vi "WILT Status Check To Turn Water On.vi"(7 "24 Hour Water Injection":i32, 8 "error in (no error)":errorcluster, 9 "Run w/o Newfi":i32, 10 "Day in":bool, 11 "Cycle Index":string) -> (0 "error out":errorcluster, 2 "Correct Cycle":bool, 3 "Day out":bool)   [LabVIEW 2016]
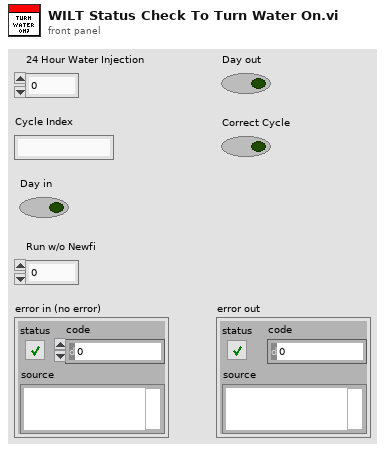
[diagram p1: front panel]
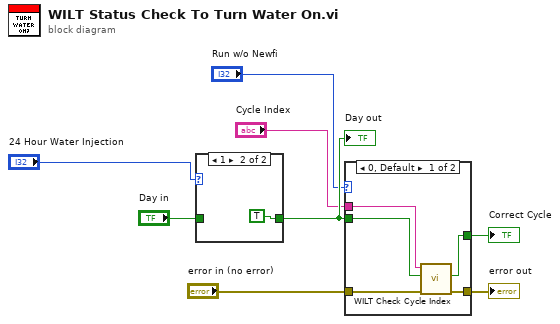
[diagram p0: block diagram]
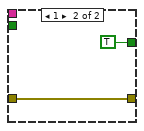
[diagram p3: hidden frame]
diagram:
  n1 = case shown="1" "24 Hour Water Injection" {
    tunnel: [w9 TRUE ("Day")] -> w7
    tunnel: "Day in" -> [w9 _]
    frame 0, Default {
    }
    frame 1 {
    }
  }
  "Day out" <- w7
  n2 = case shown="0, Default" "Run w/o Newfi" {
    tunnel: "error in (no error)" -> [w15 w17]
    tunnel: [w14 w17] -> w2
    tunnel: [w13 TRUE ("Correct Cycle")] -> w3
    tunnel: "Cycle Index" -> [w12 _]
    tunnel: w7 -> [w11 _]
    frame 0, Default {
      n3 = call "WILT Check Cycle Index.vi"("error in"=w15, "Day"=w11, "Cycle Index"=w12) -> ("error out"=w14:errorcluster, "Correct Cycle"=w13:bool)  [unwired: 7 in]
    }
    frame 1 {
    }
  }
  "Correct Cycle" <- w3
  "error out" <- w2
